vi "swabian_histogram_data.vi"(8 "error in (no error)":errorcluster, 9 "acq_time":i64 min=0, 10 "histo-settings":T1={"start_time(10^s)"=0.0, "stop_time(10^s)"=0.0, "start_channel"=enum."No Selection", "stop-channel"=enum."No Selection", "n_bins"=0, "Channels to\nHistogram"=[FALSE, FALSE, FALSE, FALSE, FALSE, FALSE, FALSE, FALSE]}, 11 "swabian_local_data":T3={"events"={"update_status"=refnum, "update_chart"=refnum, "update_xy"=refnum, "send_channel_data"=refnum}, "stop_q"=refnum, "tagger_reference"=refnum, "connect_button"=refnum, "counter_reference"=refnum, "tagger_stream_reference"=refnum, "log_reference"=refnum, "current_log_offset"=0, "tt20_buffer_q"=refnum, "stream_to_file_button"=refnum, "num_records"=0, "connected?"=FALSE, "plots"=refnum, "histogram_bin_edges"=[], "histogrammer"=refnum, "plot_lifetimes"=refnum, "xy_graph"=refnum, "Reference\nChannel"=enum."ch0"}) -> (0 "error out":errorcluster, 3 "swabian_local_data 2":T3={"events"={"update_status"=refnum, "update_chart"=refnum, "update_xy"=refnum, "send_channel_data"=refnum}, "stop_q"=refnum, "tagger_reference"=refnum, "connect_button"=refnum, "counter_reference"=refnum, "tagger_stream_reference"=refnum, "log_reference"=refnum, "current_log_offset"=0, "tt20_buffer_q"=refnum, "stream_to_file_button"=refnum, "num_records"=0, "connected?"=FALSE, "plots"=refnum, "histogram_bin_edges"=[], "histogrammer"=refnum, "plot_lifetimes"=refnum, "xy_graph"=refnum, "Reference\nChannel"=enum."ch0"})   [LabVIEW 2015]
uses:
  swabian_local_data_tdef.ctl
  swabian_events_tdef.ctl
  update_chart_tdef.ctl
  channel_data_tdef.ctl
  C:/Users/bspoka/Dropbox (MIT)/Swabian/lib/TTCSharp32.dll
  lib/TTCSharp32.dll
  swabian_buffer_tdef.ctl
  reference_checkbox_tdef.ctl
  swabian_hisotgram_settings.ctl
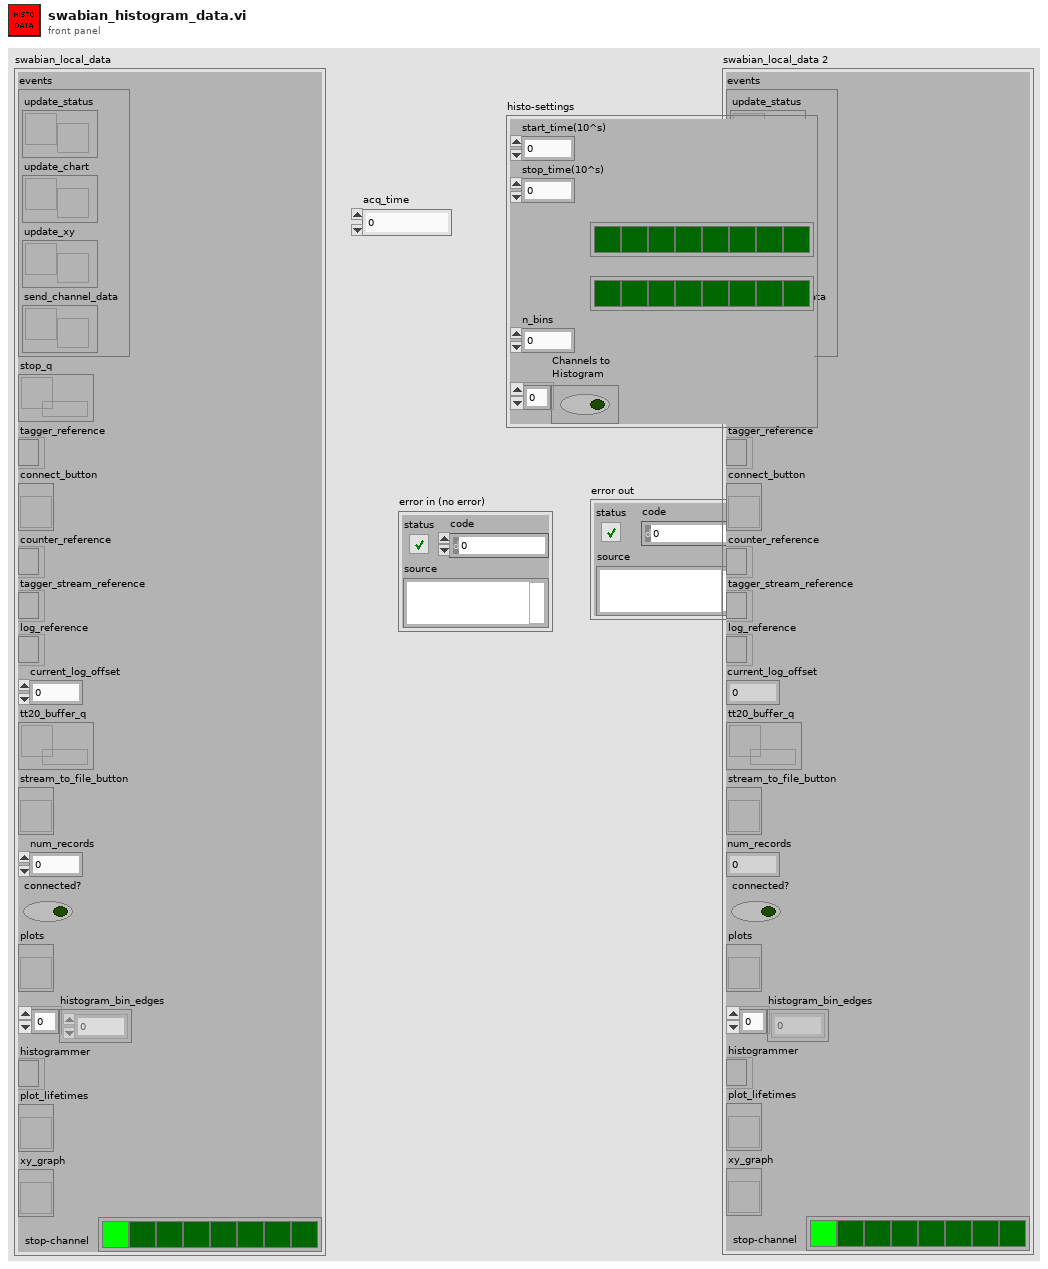
[diagram p1: front panel]
types:
  T1 = typedef "swabian_hisotgram_settings.ctl" = cluster{"start_time(10^s)":dbl, "stop_time(10^s)":dbl, "start_channel":T2, "stop-channel":T2, "n_bins":i32, "Channels to\nHistogram":bool[]}
  T2 = typedef "reference_checkbox_tdef.ctl" = enum32{"No Selection", "ch0", "ch1", "ch2", "ch3", "ch4", "ch5", "ch6", "ch7"}
  T3 = typedef "swabian_local_data_tdef.ctl" = cluster{"events":T4, "stop_q":refnum<queue>, "tagger_reference":refnum<k24>, "connect_button":refnum<vi>, "counter_reference":refnum<k24>, "tagger_stream_reference":refnum<k24>, "log_reference":refnum<file>, "current_log_offset":i64, "tt20_buffer_q":refnum<queue>, "stream_to_file_button":refnum<vi>, "num_records":u64, "connected?":bool, "plots":refnum<vi>, "histogram_bin_edges":i64[], "histogrammer":refnum<k24>, "plot_lifetimes":refnum<vi>, "xy_graph":refnum<vi>, "Reference\nChannel":T2}
  T4 = typedef "swabian_events_tdef.ctl" = cluster{"update_status":refnum<user-event>, "update_chart":refnum<user-event>, "update_xy":refnum<user-event>, "send_channel_data":refnum<user-event>}
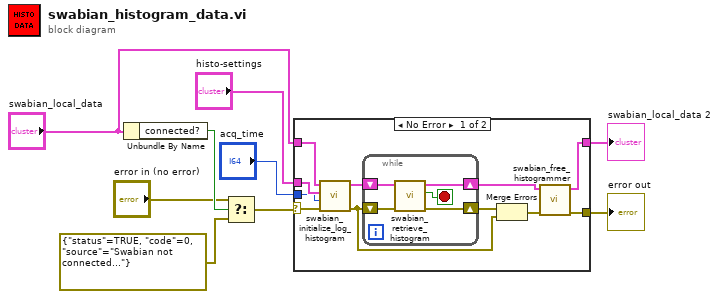
[diagram p0: block diagram]
diagram:
  n1 = Unbundle By Name("swabian_local_data") -> ("connected?"=w6:bool)
  n2 = Select(t="error in (no error)", s=w6, f=errorcluster {"status"=TRUE, "code"=0, "source"="Swabian not connected..."}) -> (s? t:f=w2:errorcluster)
  n3 = case shown="No Error" w2 {
    selector: w2 -> [w12 w26]
    tunnel: "swabian_local_data" -> [w18 w27]
    tunnel: "acq_time" -> [w15 _]
    tunnel: [w11 w26] -> w8
    tunnel: [w10 w27] -> w7
    tunnel: "histo-settings" -> [w16 _]
    frame No Error {
      n4 = call "swabian_initialize_log_histogram.vi"("error in (no error)"=w12, "acq_time"=w15, "histo-settings"=w16, "swabian_local_data"=w18) -> ("error out"=w19:errorcluster, "swabian_local_data 2"=w17:T3)  [unwired: 6 in]
      n5 = while {
        shift-right: [w21] -> w20
        shift-left: w19 -> [w25]
        shift-right: [w22] -> w13
        shift-left: w17 -> [w23]
        stop <- w24 stop-if-true
        n6 = call "swabian_retrieve_histogram.vi"("error in (no error)"=w25, "swabian_local_data"=w23) -> ("error out"=w21:errorcluster, "stop"=w24:bool, "swabian_local_data 2"=w22:T3)  [unwired: 7 in]
      }
      n7 = Merge Errors(w20, w19) -> (w14:errorcluster)
      n8 = call "swabian_free_histogrammer.vi"("error in (no error)"=w14, "swabian_local_data"=w13) -> ("error out"=w11:errorcluster, "swabian_local_data 2"=w10:T3)  [unwired: 8 in]
    }
    frame Error {
    }
  }
  "swabian_local_data 2" <- w7
  "error out" <- w8
